vi "Sistema de ventilación_V2.vi"() -> ()   [LabVIEW 2023]
uses:
  <vilib>/MakerHub/LINX/Public/Peripherals/Analog/Analog Read 1 Chan.vi
  <vilib>/MakerHub/LINX/Public/Peripherals/Digital/Digital Write 1 Chan.vi
  <vilib>/MakerHub/LINX/Public/Peripherals/Analog/Analog Read N Chans.vi
  <vilib>/MakerHub/LINX/Public/Peripherals/Digital/Digital Write N Chans.vi
  <vilib>/MakerHub/LINX/Private/Local IO/LinxAnalogRead.vi
  <vilib>/MakerHub/LINX/Public/Utilities/Check Channel.vi
  <vilib>/MakerHub/LINX/Private/Local IO/LinxDigitalWrite.vi
  <vilib>/MakerHub/LINX/Public/Utilities/Open Serial.vi
  <vilib>/MakerHub/LINX/Public/Sensors/Motion/Servo/Servo Open One Channel.vi
  <vilib>/MakerHub/LINX/Public/Peripherals/Analog/Analog Write 1 Chan.vi
  <vilib>/MakerHub/LINX/Private/Utilties/Generate Error.vi
  <vilib>/MakerHub/LINX/Public/Sensors/Temperature/TMP3x/TMP35.vi
  <vilib>/MakerHub/LINX/Public/Sensors/Motion/Servo/Servo Set Pulse Width One Channel.vi
  <vilib>/MakerHub/LINX/Public/Sensors/Motion/Servo/Servo Close One Channel.vi
  <vilib>/MakerHub/LINX/LMH-LINX.lvlib
  <vilib>/MakerHub/LINX/Public/Sensors/Temperature/TMP3x/TMP3x.lvlib
  <vilib>/MakerHub/LINX/Public/Sensors/Motion/Servo/Servo.lvlib
panel:
  out "?":bool
  out "?":bool
  out "?":bool
  out "?":bool
  in  "?":bool
  out "Serevo Aire Angulo":string
  out "Serevo Temp Angulo":string
  in  "Serial Port":refnum<visa-resource-name>
  out "?":bool
  out "?":bool
  out "?":bool
  out "?":bool
  out "?":bool
  out "?":bool
  out "?":bool
  out "?":bool
  out "?":bool
  out "?":bool
  out "?":bool
  out "?":bool
  out "?":bool
  out "?":bool
  out "?":bool
  out "?":bool
  out "?":bool
  out "?":bool
  in  "?":bool
  out "Filtro de Calor":bool
  out "Filtro de Aire":bool
  out "Calidad del aire":dbl(knob) scale=0.0..1800.0
  out "Temperatura":dbl(slide) scale=0.0..60.0
  out "t [sec]":dbl
  out "Iteration No":i32
  in  "?":bool
  out "VI is running?":bool caption="ON/OFF"
  # "SISTEMA DE VENTILACIÓN DE DOBLE FLUJO"
  # "Entrada"
  # "Salida"
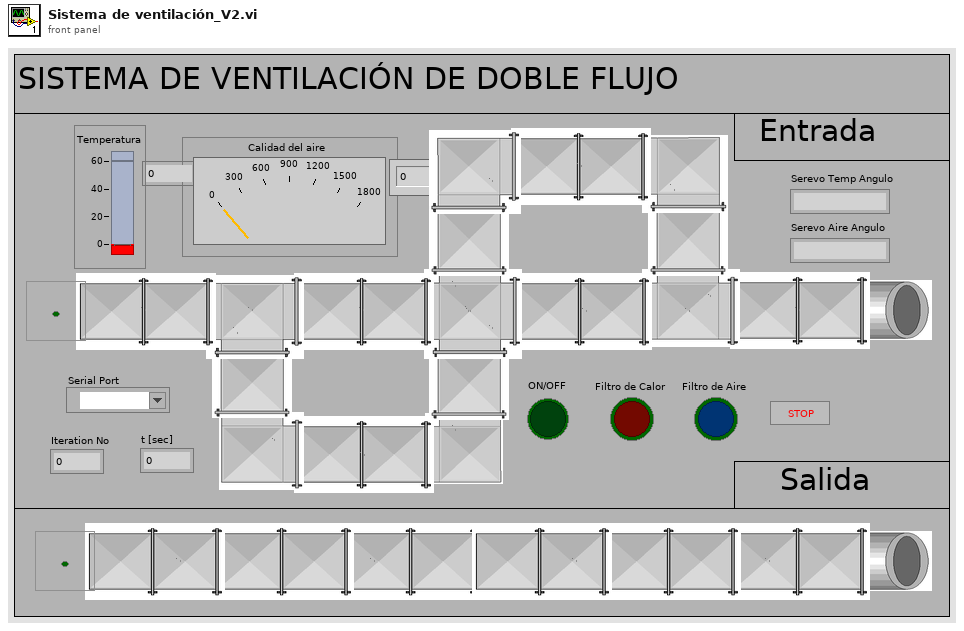
[diagram p1: front panel]
types:
  T1 = typedef "LMH-LINX.lvlib/LINX Ref.ctl" = cluster{"IO":T2, "Interface":T3, "LINX Device Config":T4}
  T2 = typedef "LMH-LINX.lvlib/Platform.ctl" = enum16{"Remote", "Local"}
  T3 = typedef "LMH-LINX.lvlib/Interface.ctl" = enum16{"Serial", "TCP"}
  T4 = typedef "LMH-LINX.lvlib/Device.lvlib/LINX Device Config.ctl" = cluster{"Interface":T3, "COM Port":refnum<visa-resource-name>, "TCP Configuration":T5, "Device Family":u8, "Device ID":u8, "Device Name":string, "TCP Ref":refnum<k5>, "Channels":T6}
  T5 = typedef "LMH-LINX.lvlib/Device.lvlib/TCP Config.ctl" = cluster{"IP Address":string, "Port":u16}
  T6 = typedef "LMH-LINX.lvlib/Channels.ctl" = cluster{"DI":u8[], "DO":u8[], "AI":u8[], "AO":u8[], "PWM":u8[], "QE":u8[], "UART":u8[], "I2C 2":u8[], "SPI":u8[], "CAN":u8[], "Servo":u8[], "AI Ref (V)":dbl, "AI Resolution (Bits)":u8, "AO Ref (V)":dbl, "AO Resolution (Bits)":u8}
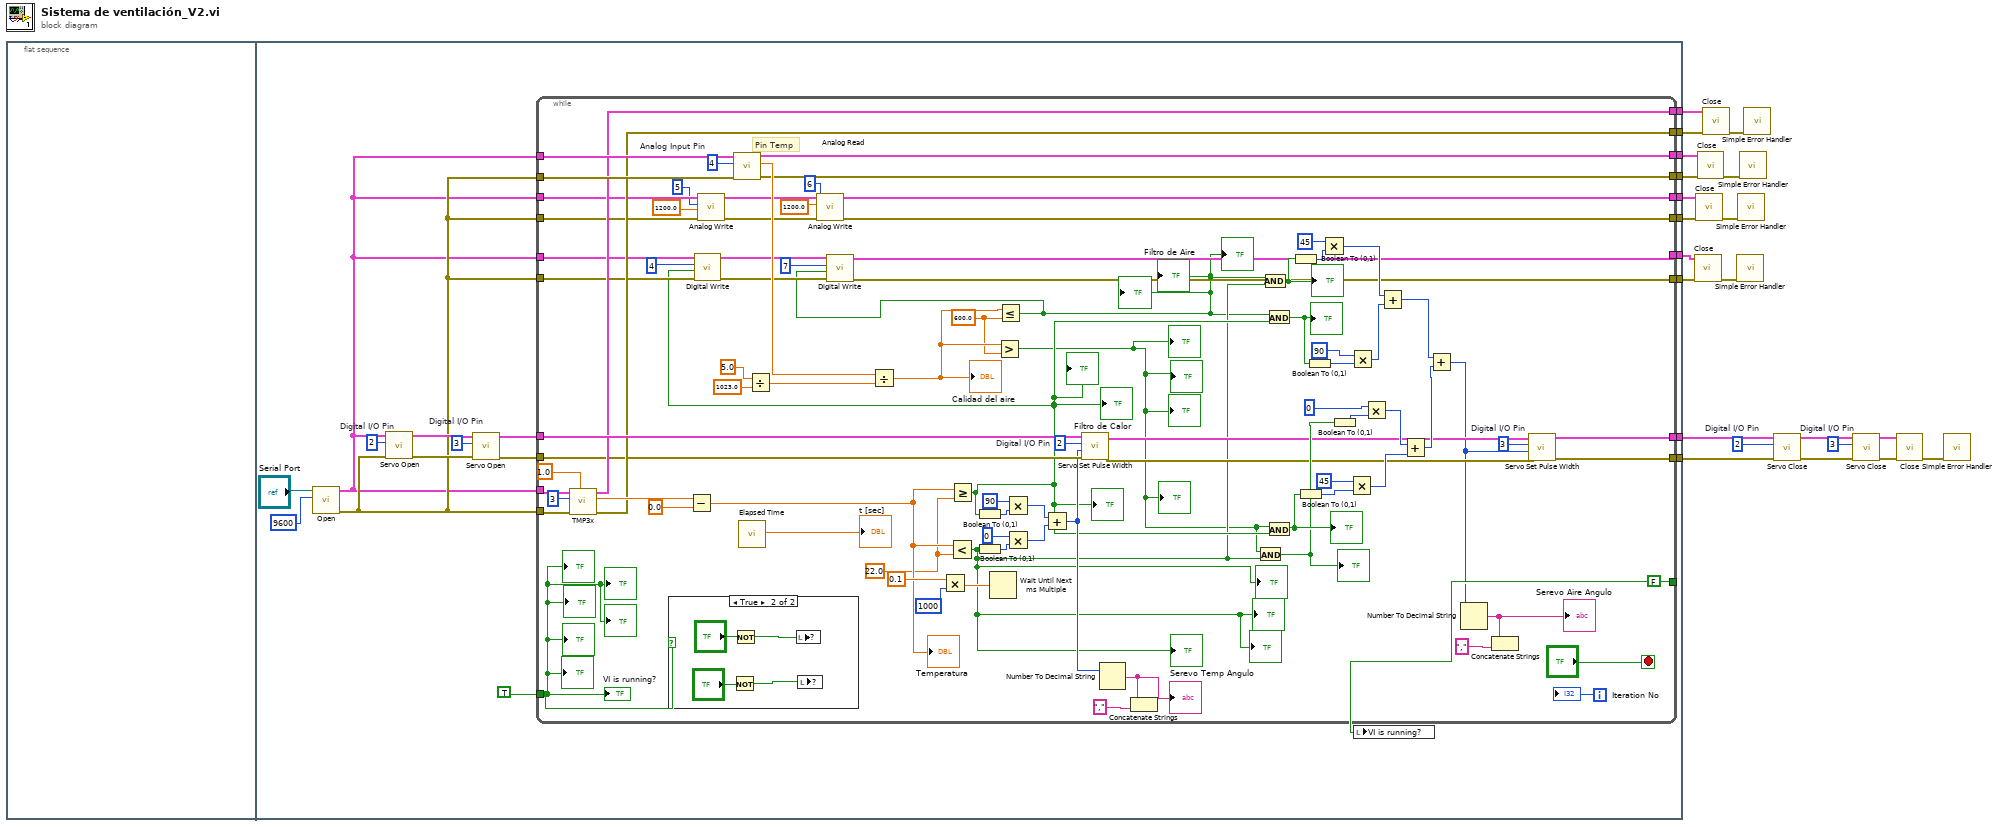
[diagram p0: block diagram]
diagram:
  w12 = 3  # Digital I/O Pin
  w13 = 2  # Digital I/O Pin
  n1 = flat-sequence {
    tunnel: [w40] -> w21
    tunnel: [w38] -> w19
    tunnel: [w37] -> w17
    tunnel: [w36] -> w16
    tunnel: [w35] -> w15
    tunnel: [w34] -> w14
    tunnel: [w27] -> w5
    tunnel: [w26] -> w4
    tunnel: [w23] -> w2
    tunnel: [w22] -> w1
    frame #0 {
    }
    frame #1 {
      w32 = 3  # Digital I/O Pin
      w33 = 2  # Digital I/O Pin
      n2 = call-poly <vilib>:"Open.vi"("Baud Rate Override"=u32 9600, "Serial Port"="Serial Port") -> ("Error Out"=w25:errorcluster, "LINX Resource"=w24:T1)  [unwired: 7 in, 1 out]
      n3 = call-poly <vilib>:"Servo Open.vi"("Error In"=w25, "Servo Channel"=w33, "LINX Resource"=w24) -> ("Error Out"=w31:errorcluster, "LINX Resource"=w29:T1)  [unwired: 7 in]
      n4 = call-poly <vilib>:"Servo Open.vi"("Error In"=w31, "Servo Channel"=w32, "LINX Resource"=w29) -> ("Error Out"=w30:errorcluster, "LINX Resource"=w28:T1)  [unwired: 7 in]
      n5 = while {
        tunnel: [FALSE] -> w42
        tunnel: TRUE -> [w60]
        tunnel: w24 -> [w125]
        tunnel: [w86] -> w40
        tunnel: w25 -> [w123]
        tunnel: w24 -> [w120]
        tunnel: [w87] -> w38
        tunnel: w25 -> [w115]
        tunnel: [w80] -> w37
        tunnel: [w79] -> w36
        tunnel: w28 -> [w88]
        tunnel: w30 -> [w85]
        tunnel: [w82] -> w35
        tunnel: [w81] -> w34
        tunnel: w25 -> [w76]
        tunnel: w24 -> [w75]
        tunnel: [w68] -> w27
        tunnel: [w67] -> w26
        tunnel: w25 -> [w59]
        tunnel: w24 -> [w58]
        tunnel: [w53] -> w23
        tunnel: [w52] -> w22
        i -> [w127]
        stop <- "?" stop-if-true
        w84 = 2  # Digital I/O Pin
        w77 = 3  # Digital I/O Pin
        w114 = 4  # Analog Input Pin
        w50 = 600.0
        w48 = 22.0
        # "Pin Temp"
        n6 = call-poly <vilib>:"TMP3x.vi"("Analog Ref Override"=1.0, "Error In"=w123, "Analog Channel"=3, "LINX Resource"=w125) -> ("Error Out"=w87:errorcluster, "Temp C"=w121:dbl, "LINX Resource"=w86:T1)  [unwired: 5 in]
        n7 = case shown="True" w60 {
          frame False {
          }
          frame True {
            n8 = Not(x="?") -> (.not. x?=w133:bool)
            n9 = Not(x="?") -> (.not. x?=w135:bool)
            n10 = local write item#8(w135) -> ()
            n11 = local write item#30(w133) -> ()
          }
        }
        n12 = Subtract(x=w121, y=0.0) -> (x-y=w49:dbl)
        "Temperatura" <- w49
        n13 = call-poly <vilib>:"Analog Write.vi"("Error In"=w76, "AO Value"=1200.0, "AO Channel"=5, "LINX Resource"=w75) -> ("Error Out"=w69:errorcluster, "LINX Resource"=w70:T1)  [unwired: 6 in]
        n14 = call-poly <vilib>:"Analog Read.vi"("Error In"=w115, "Analog Channel"=w114, "LINX Resource"=w120) -> ("Error Out"=w79:errorcluster, "Voltage"=w117:dbl, "LINX Resource"=w80:T1)  [unwired: 5 in, 1 out]
        n15 = call "Elapsed Time"() -> ("Elapsed Time (s)"=→"t [sec]":dbl)  [unwired: 12 in, 7 out]
        n16 = Divide(x=5.0, y=1023.0) -> (x/y=w116:dbl)
        n17 = call-poly <vilib>:"Analog Write.vi"("Error In"=w69, "AO Value"=1200.0, "AO Channel"=6, "LINX Resource"=w70) -> ("Error Out"=w68:errorcluster, "LINX Resource"=w67:T1)  [unwired: 6 in]
        n18 = Divide(x=w117, y=w116) -> (x/y=w51:dbl)
        "Calidad del aire" <- w51
        n19 = Multiply(x=0.1, y=1000) -> (x*y=w130:dbl)
        n20 = Less?(x=w49, y=w48) -> (x < y?=w46:bool)
        "?" <- w46
        "?" <- w46
        "?" <- w46
        "?" <- w46
        n21 = Greater Or Equal?(x=w49, y=w48) -> (x >= y?=w47:bool)
        "Filtro de Calor" <- w47
        "?" <- w47
        "?" <- w47
        n22 = call-poly <vilib>:"Digital Write.vi"("Error In"=w59, "Output Value"=w47, "DO Channel"=4, "LINX Resource"=w58) -> ("Error Out"=w54:errorcluster, "LINX Resource"=w55:T1)  [unwired: 6 in]
        n23 = Boolean To (0,1)(Boolean=w47) -> (0, 1=w93:i16)
        n24 = Boolean To (0,1)(Boolean=w46) -> (0, 1=w91:i16)
        n25 = Wait Until Next ms Multiple(millisecond multiple=w130) -> ()  [unwired: 1 out]
        n26 = Greater?(x=w51, y=w50) -> (0:w45:bool)
        "?" <- w45
        "?" <- w45
        "?" <- w45
        "?" <- w45
        n27 = Less Or Equal?(x=w51, y=w50) -> (x <= y?=w44:bool)
        "Filtro de Aire" <- w44
        "?" <- w44
        "?" <- w44
        n28 = call-poly <vilib>:"Digital Write.vi"("Error In"=w54, "Output Value"=w44, "DO Channel"=7, "LINX Resource"=w55) -> ("Error Out"=w52:errorcluster, "LINX Resource"=w53:T1)  [unwired: 6 in]
        n29 = Multiply(x=90, y=w93) -> (x*y=w89:i32)
        n30 = Multiply(x=0, y=w91) -> (x*y=w90:i32)
        n31 = Add(x=w89, y=w90) -> (x+y=w64:i32)
        n32 = call-poly <vilib>:"Servo Set Pulse Width.vi"("Error In"=w85, "Pulse Width (uS)"=w64, "Servo Channel"=w84, "LINX Resource"=w88) -> ("Error Out"=w83:errorcluster, "LINX Resource"=w78:T1)  [unwired: 6 in]
        n33 = Number To Decimal String(number=w64) -> (decimal integer string=w66:string)  [unwired: 1 in]
        "Serevo Temp Angulo" <- w66
        n34 = Concatenate Strings(w66, "," ("string")) -> ()  [unwired: 1 out]
        n35 = And(x=w45, y=w46) -> (x .and. y?=w104:bool)
        "?" <- w104
        n36 = And(x=w44, y=w46) -> (x .and. y?=w111:bool)
        "?" <- w111
        n37 = And(x=w44, y=w47) -> (x .and. y?=w101:bool)
        "?" <- w101
        n38 = And(x=w45, y=w47) -> (x .and. y?=w107:bool)
        "?" <- w107
        n39 = Boolean To (0,1)(Boolean=w111) -> (0, 1=w110:i16)
        n40 = Boolean To (0,1)(Boolean=w107) -> (0, 1=w108:i16)
        n41 = Boolean To (0,1)(Boolean=w101) -> (0, 1=w102:i16)
        n42 = Multiply(x=45, y=w110) -> (x*y=w100:i32)
        n43 = Boolean To (0,1)(Boolean=w104) -> (0, 1=w105:i16)
        n44 = Multiply(x=45, y=w108) -> (x*y=w97:i32)
        n45 = Multiply(x=90, y=w102) -> (x*y=w99:i32)
        n46 = Multiply(x=0, y=w105) -> (x*y=w98:i32)
        n47 = Add(x=w100, y=w99) -> (x+y=w95:i32)
        n48 = Add(x=w97, y=w98) -> (x+y=w96:i32)
        n49 = Add(x=w95, y=w96) -> (x+y=w61:i32)
        n50 = Number To Decimal String(number=w61) -> (decimal integer string=w63:string)  [unwired: 1 in]
        "Serevo Aire Angulo" <- w63
        n51 = Concatenate Strings(w63, "," ("string")) -> ()  [unwired: 1 out]
        n52 = call-poly <vilib>:"Servo Set Pulse Width.vi"("Error In"=w83, "Pulse Width (uS)"=w61, "Servo Channel"=w77, "LINX Resource"=w78) -> ("Error Out"=w81:errorcluster, "LINX Resource"=w82:T1)  [unwired: 6 in]
        "VI is running?" <- w60
        "Iteration No" <- w127
        "?" <- w60
        "?" <- w60
        "?" <- w60
        "?" <- w60
        "?" <- w60
        "?" <- w60
      }
      n53 = local write "VI is running?"(w42) -> ()
    }
  }
  n54 = call <vilib>:"Close.vi"("Error In"=w1, "LINX Resource"=w2) -> ("Error Out"=w3:errorcluster)  [unwired: 9 in]
  n55 = call <vilib>:"Close.vi"("Error In"=w5, "LINX Resource"=w4) -> ("Error Out"=w6:errorcluster)  [unwired: 9 in]
  n56 = call <vilib>:"Close.vi"("Error In"=w16, "LINX Resource"=w17) -> ("Error Out"=w18:errorcluster)  [unwired: 9 in]
  n57 = call <vilib>:"Close.vi"("Error In"=w19, "LINX Resource"=w21) -> ("Error Out"=w20:errorcluster)  [unwired: 9 in]
  n58 = call <vilib>:"Simple Error Handler.vi"("error in (no error)"=w3) -> ()  [unwired: 4 in, 5 out]
  n59 = call <vilib>:"Simple Error Handler.vi"("error in (no error)"=w6) -> ()  [unwired: 4 in, 5 out]
  n60 = call <vilib>:"Simple Error Handler.vi"("error in (no error)"=w18) -> ()  [unwired: 4 in, 5 out]
  n61 = call <vilib>:"Simple Error Handler.vi"("error in (no error)"=w20) -> ()  [unwired: 4 in, 5 out]
  n62 = call-poly <vilib>:"Servo Close.vi"("Error In"=w14, "Servo Channel"=w13, "LINX Resource"=w15) -> ("Error Out"=w9:errorcluster, "LINX Resource"=w11:T1)  [unwired: 7 in]
  n63 = call-poly <vilib>:"Servo Close.vi"("Error In"=w9, "Servo Channel"=w12, "LINX Resource"=w11) -> ("Error Out"=w8:errorcluster, "LINX Resource"=w10:T1)  [unwired: 7 in]
  n64 = call <vilib>:"Close.vi"("Error In"=w8, "LINX Resource"=w10) -> ("Error Out"=w7:errorcluster)  [unwired: 9 in]
  n65 = call <vilib>:"Simple Error Handler.vi"("error in (no error)"=w7) -> ()  [unwired: 4 in, 5 out]
